vi "Determine Multiplier Value.vi"(2 "mult color":T1) -> (6 "multiplier":dbl format="%_3p")   [LabVIEW 2018]
doc: "Determines the numerical multiplier value corresponding to the selected resistor multiplier color.\n\nThe VI receives the Multiplier Color Enum value and uses it as an index into the exponent array provided by the Exponents--constant.vi.\n\nThe <b>exponents--constant.vi</b> contains the following exponent array:\n\n[-2, -1, 0, 1, 2, 3, 4, 5, 6, 7, 8, 9]\n\nThe Enum value is used as the array index. The selected exponent is then converted to the corresponding multiplier value using 10^x.\n\nThe resistor color code mapping is:\n\nSilver -> 10^(-2)\nGold -> 10^(-1)\nBlack -> 10^(0)\nBrown -> 10^(1)\nRed -> 10^(2)\nOrange -> 10^(3)\nYellow -> 10^(4)\nGreen -> 10^(5)\nBlue -> 10^(6)\nViolet -> 10^(7)\nGrey -> 10^(8)\nWhite -> 10^(9)"
uses:
  multiplier--enum.ctl
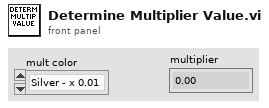
[diagram p1: front panel]
types:
  T1 = typedef "multiplier--enum.ctl" = enum16{"Silver - x 0.01", "Gold - x 0.1 ", "Black - x 1", "Brown - x 10", "Red - x 100", "Orange - x 1k", "Yellow - x 10k", "Green - 100k", "Blue - x 1M", "Violet - x10 M", "Grey - x 100M", "White - x 1G"}
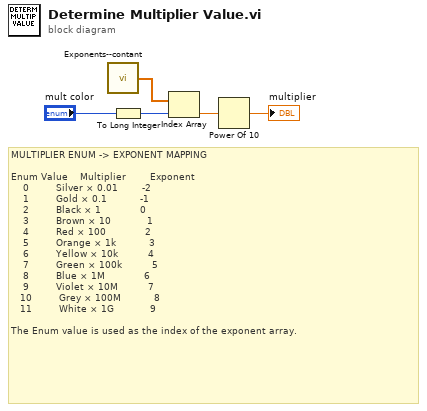
[diagram p0: block diagram]
diagram:
  # "MULTIPLIER ENUM -> EXPONENT MAPPING\n\nEnum Value    Multiplier        Exponent\n    0         Silver × 0.01        -2\n    1         Gold × 0.1           -1\n    2         Black × 1             0\n    3         Brown × 10            1\n    4         Red × 100             2\n    5         Orange × 1k           3\n    6         Yellow × 10k          4\n    7         Green × 100k          5\n    8         Blue × 1M             6\n    9         Violet × 10M          7\n   10         Grey × 100M           8\n   11         White × 1G            9\n\nThe Enum value is used as the index of the exponent array."
  n1 = call "Exponents--contant.vi"() -> ("exponent"=w3:dbl[])  [unwired: 6 in]
  n2 = To Long Integer(number="mult color") -> (32bit integer=w4:i32)
  n3 = Index Array(array=w3, index=w4) -> (element=w2:dbl)
  n4 = Power Of 10(x=w2) -> (10^x=→"multiplier":dbl)
